vi "GamePlayfield_CheckPerfectClear.vi"(2 "Player":u8) -> (16 "PerfectClear":bool)   [LabVIEW 2018]
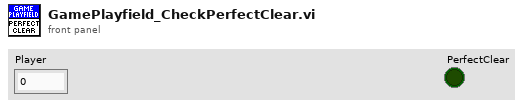
[diagram p1: front panel]
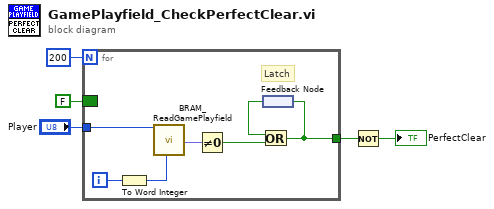
[diagram p0: block diagram]
diagram:
  n1 = for {
    N: 200 -> [_]
    tunnel: "Player" -> [w11]
    border: FALSE -> [_]
    tunnel: [w7] -> w1
    i -> [w10]
    # "Latch"
    n2 = To Word Integer(number=w10) -> (16bit integer=w9:i16)
    n3 = call "BRAM_ReadGamePlayfield.vi"("Player IN"=w11, "Address"=w9) -> ("Data"=w12:fxp<+,3,3>)  [unwired: 16 in, 1 out]
    n4 = Not Equal To 0?(x=w12) -> (x != 0?=w8:bool)
    n5 = feedback #1() -> (w6:bool)
    n6 = Or(x=w6, y=w8) -> (x .or. y?=w7:bool)
    n7 = feedback-in #1(w7) -> ()
  }
  n8 = Not(x=w1) -> (.not. x?=→"PerfectClear":bool)
